vi "LSTM_Demo.vi"() -> ()   [LabVIEW 2014]
uses:
  <vilib>/Analysis/Matrix/Datatypes/RealMatrix.ctl
  <vilib>/Analysis/Matrix/NI_Matrix.lvlib
panel:
  in  "x[t]":T1=[[0.0], [1.0], [0.0]]
  in  "c[t-1]":T1=[[0.5], [0.5]] format="%.2f"
  in  "h[t-1]":T1=[[0.3], [0.7]] format="%.2f"
  out "param clusters":T2={"input weights"={"Wx[N,M]"=[[0.9438476798368013, -0.2588511705719912, -1.5636057855464167], [-0.522971075467345, -0.23863700075182345, -0.34173596041915355]], "Wh[M,M]"=[[1.5843729928280075, -0.23959132310096362], [0.6242601180113263, 0.7651884613133993]], "Wc[M,M]"=[[1.1467599184133548, -1.2337055595382362], [-1.118839443009057, -1.081335469619707]], "bias"=[[0.029310921526310665], [-0.6167118014447182]]}, "candidate weights"={"Wx[N,M]"=[[1.394919980619541, -1.3602645113484602, 0.9702458857095743], [-0.7935507680500221, -0.12746010642691252, 0.41484005460882545]], "Wh[M,M]"=[[0.6658037071872467, 0.6725629007945276], [0.005239171448543704, 2.8731284987889167]], "bias"=[[0.23924878282513978], [-1.7402343708405232]]}, "forget weights"={"Wx[N,M]"=[[-1.0289474610577152, 0.6992203301677954, 0.1925136059426792], [1.7831316574336573, 2.0050616884014425, 0.6941532067697257]], "Wh[M,M]"=[[1.007185750636882, -0.47231783611022177], [0.5347300718547148, 0.531151284650078]], "Wc[M,M]"=[[0.3984996876854651, -0.7543369418916427], [-2.2749329665806575, -1.4202017205007216]], "bias"=[[-0.15830276336997642], [-1.574835827064872]]}, "output weights"={"Wx[N,M]"=[[-0.2776764592286954, 0.14979950706786388, -1.613593199175164], [-0.3082351227161497, 1.3560431033826263, -0.04571416818624348]], "Wh[M,M]"=[[1.0897324168036, 1.1342464539277195], [-1.3557197503994423, -1.2995675832305424]], "Wc[M,M]"=[[1.115929626042798, 1.2784532838922105], [-2.055332842692169, -1.1763839750933645]], "bias"=[[-0.26761779907665134], [0.8943334871365315]]}} {"input weights"."Wx[N,M]" format="%.2g"; "input weights"."Wh[M,M]" format="%.2g"; "input weights"."Wc[M,M]" format="%.2g"; "input weights"."bias" format="%.2g"; "candidate weights"."Wx[N,M]" format="%.2g"; "candidate weights"."Wh[M,M]" format="%.2g"; "candidate weights"."bias" format="%.2g"; "forget weights"."Wx[N,M]" format="%.2g"; "forget weights"."Wh[M,M]" format="%.2g"; "forget weights"."Wc[M,M]" format="%.2g"; "forget weights"."bias" format="%.2g"; "output weights"."Wx[N,M]" format="%.2g"; "output weights"."Wh[M,M]" format="%.2g"; "output weights"."Wc[M,M]" format="%.2g"; "output weights"."bias" format="%.2g"}
  out "h[t]":T1=[[0.11924558384048108], [0.9291561164037933]] format="%.2f"
  out "c[t]":T1=[[0.11924558384048108], [0.9291561164037933]] format="%.2f"
  in  "M":u64=2
  in  "N":u64=2
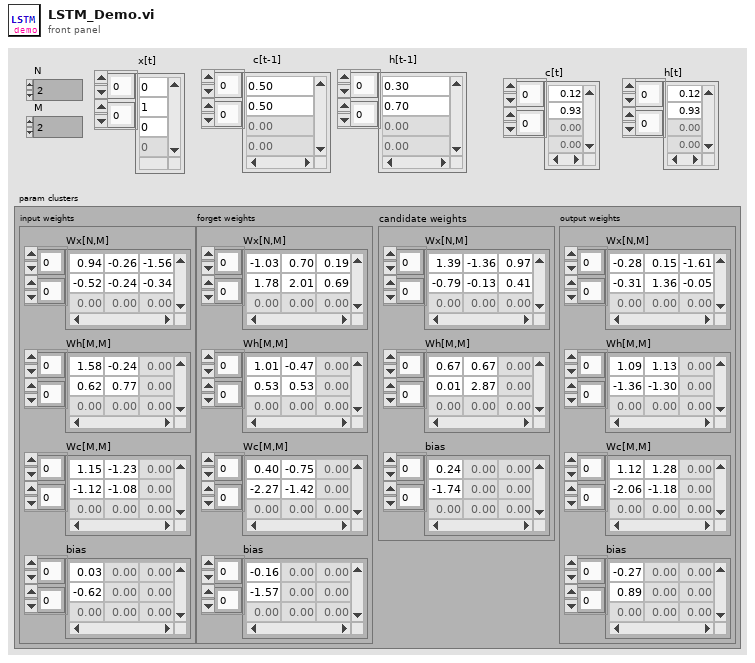
[diagram p1: front panel]
types:
  T1 = typedef "NI_Matrix.lvlib/RealMatrix.ctl" = dbl[][]
  T2 = cluster{"input weights":cluster{"Wx[N,M]":T1, "Wh[M,M]":T1, "Wc[M,M]":T1, "bias":T1}, "candidate weights":cluster{"Wx[N,M]":T1, "Wh[M,M]":T1, "bias":T1}, "forget weights":cluster{"Wx[N,M]":T1, "Wh[M,M]":T1, "Wc[M,M]":T1, "bias":T1}, "output weights":cluster{"Wx[N,M]":T1, "Wh[M,M]":T1, "Wc[M,M]":T1, "bias":T1}}
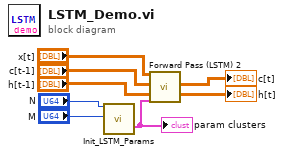
[diagram p0: block diagram]
diagram:
  n1 = call "Init_LSTM_Params.vi"("Dimension"="N", "Hidden Layers"="M") -> ("param clusters"=w8:T2)  [unwired: 17 in]
  "param clusters" <- w8
  n2 = call "Forward Pass (LSTM) 2.vi"("x[t]"="x[t]", "c[t-1]"="c[t-1]", "h[t-1]"="h[t-1]", "param clusters"=w8) -> ("c[t]"=→"c[t]":T1, "h[t]"=→"h[t]":T1)  [unwired: 14 in]
